vi "VisionX-1LOOP-Main.vi"(8 "ErrI":errorcluster) -> (0 "ErrO":errorcluster)   [LabVIEW 2020]
uses:
  <vilib>/vision/Measure.llb/Straight Edge Options.ctl
  <vilib>/vision/Measure.llb/Straight Edge Process.ctl
  <vilib>/vision/Image Controls.llb/IMAQ Image.ctl
  <vilib>/vision/Measure.llb/Edge Options.ctl
  <vilib>/vision/Measure.llb/Edge Polarity.ctl
  <vilib>/vision/NI_Vision_Development_Module.lvlib
panel:
  out "Pass?":bool
  out "Liquied Level":dbl format="%.2f"
  in  "Line Fit Options":T1={"Number of Lines"=1, "Type"=enum."Best Edge Rake", "Min. Score"=10.0, "Max. Score"=1000.0, "Orientation"=0.0, "Angle Range"=45.0, "Angle Tolerance"=1.0, "Step Size"=7, "Min. SNR (db)"=0.0, "Min. Points (%)"=25.0, "Hough Iterations"=5} {"Min. Points (%)" min=0.0 max=100.0; "Min. SNR (db)" min=0.0; "Max. Score" min=0.0 max=1024.0; "Min. Score" min=0.0 max=1024.0 step=1.0}
  out "Image":T3(plugin-control)
  in  "Next":bool
  in  "Exit":bool
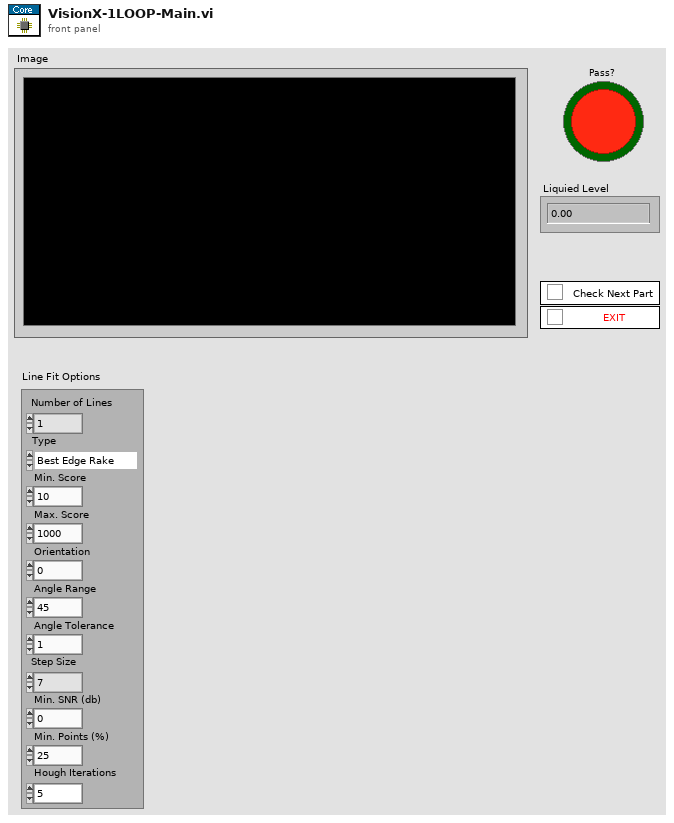
[diagram p1: front panel]
types:
  T1 = typedef "Straight Edge Options.ctl" = cluster{"Number of Lines":i32, "Type":T2, "Min. Score":dbl, "Max. Score":dbl, "Orientation":dbl, "Angle Range":dbl, "Angle Tolerance":dbl, "Step Size":u32, "Min. SNR (db)":dbl, "Min. Points (%)":dbl, "Hough Iterations":i32}
  T2 = typedef "Straight Edge Process.ctl" = enum32{"First Edge Rake", "Best Edge Rake", "Hough Edge Rake", "First Edge Projection", "Best Edge Projection"}
  T3 = typedef "IMAQ Image.ctl" = refnum<image>
  T4 = typedef "IMAQ Rectangle" = cluster{"Left":i32, "Top":i32, "Right":i32, "Bottom":i32, "Rotation":dbl}
  T5 = cluster{"Point1":cluster{"X":sgl, "Y":sgl}, "Point2":cluster{"X":sgl, "Y":sgl}}
  T6 = typedef "IMAQ Coordinate System" = cluster{"Reference System":cluster{"Origin":cluster{"X":sgl, "Y":sgl}, "Angle (deg)":sgl, "Axis Reference":u32}, "Measurement System":cluster{"Origin":cluster{"X":sgl, "Y":sgl}, "Angle (deg)":sgl, "Axis Reference":u32}}
  T7 = cluster{"Src":T3, "Dst":T3, "Parts":string[], "RefCoord":T6, "MsrCoord":T6, "MsrROI":T4, "RefLine":cluster{"Point1":cluster{"X":sgl, "Y":sgl}, "Point2":cluster{"X":sgl, "Y":sgl}}}
  T8 = typedef "Edge Options.ctl" = cluster{"Edge Polarity":T9, "Kernel Size":u32, "Width":u32, "Minimum Edge Strength":sgl, "Interpolation Type":enum32{"Zero Order", "Bilinear", "Quadratic", "Cubic", "Bilinear Fixed"}, "Data Processing Method":enum32{"Average", "Median"}}
  T9 = typedef "Edge Polarity.ctl" = u32
  T10 = cluster{"Direction":u16, "Primary Edge Options":T8, "Secondary Edge Options":T8, "Show Search Area":bool, "Show Search Lines":bool, "Show Edges Found":bool, "Show Result":bool, "Search Area Color":u32, "Search Lines Color":u32, "Edge Locations Color":u32, "Result Color":u32, "Overlay Group Name":string}
  T11 = typedef "ROI Descriptor" = cluster{"Global Rectangle":i32[], "Contours":cluster{"ID":enum32{"External", "Internal"}, "Type":u32, "Coordinates":i32[]}[]}
  T12 = cluster{"Search Direction":u32, "Edge Options":T8, "Show Search Area":bool, "Show Search Lines":bool, "Show Edges Found":bool, "Show Result":bool, "Search Area Color":u32, "Search Lines Color":u32, "Edge Locations Color":u32, "Result Color":u32, "Overlay Group Name":string}
  T13 = cluster{"Point1 (Pixels)":cluster{"X":sgl, "Y":sgl}, "Point2 (Pixels)":cluster{"X":sgl, "Y":sgl}, "Point1 (Real-World)":cluster{"X":sgl, "Y":sgl}, "Point2 (Real-World)":cluster{"X":sgl, "Y":sgl}, "Angle (Pixel)":dbl, "Angle (Real-World)":dbl, "Score":dbl, "Straightness":dbl, "Average SNR (db)":dbl, "Calibration Valid":bool}[]
  T14 = cluster{"Point1 (Pixels)":cluster{"X":sgl, "Y":sgl}, "Point2 (Pixels)":cluster{"X":sgl, "Y":sgl}, "Point1 (Real-World)":cluster{"X":sgl, "Y":sgl}, "Point2 (Real-World)":cluster{"X":sgl, "Y":sgl}, "Angle (Pixel)":dbl, "Angle (Real-World)":dbl, "Score":dbl, "Straightness":dbl, "Average SNR (db)":dbl, "Calibration Valid":bool}
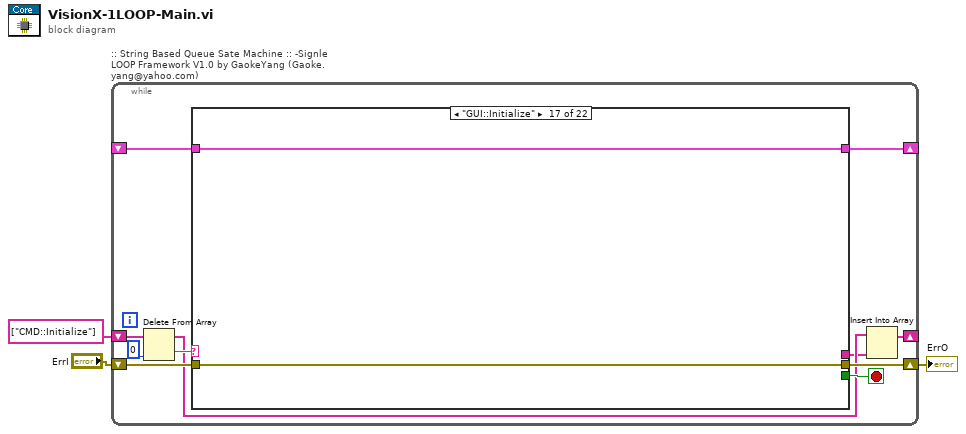
[diagram p0: block diagram]
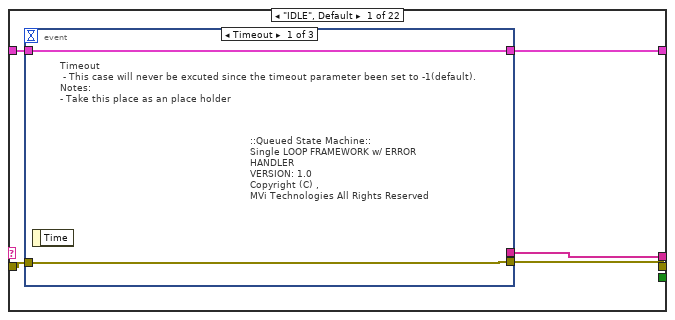
[diagram p2: hidden frame]
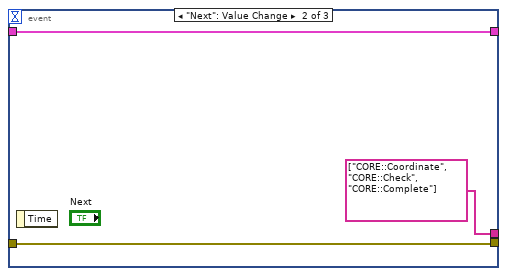
[diagram p3: hidden frame]
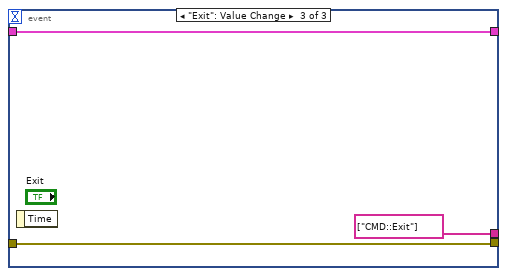
[diagram p4: hidden frame]
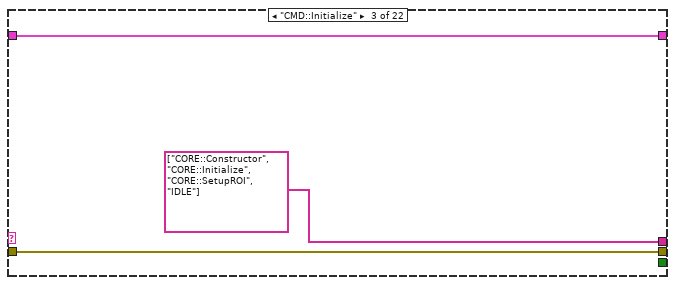
[diagram p6: hidden frame]
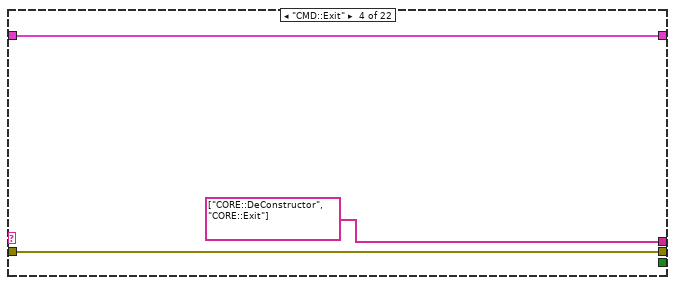
[diagram p7: hidden frame]
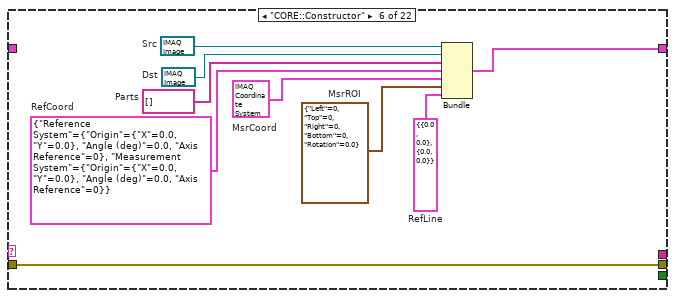
[diagram p9: hidden frame]
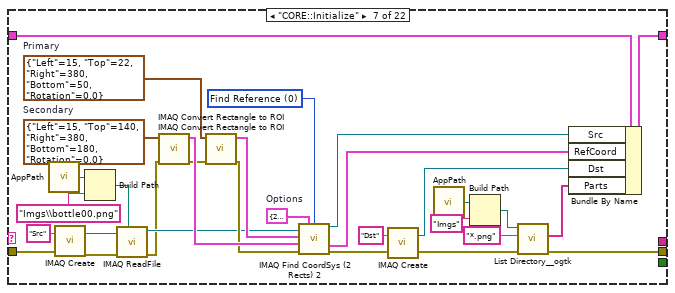
[diagram p10: hidden frame]
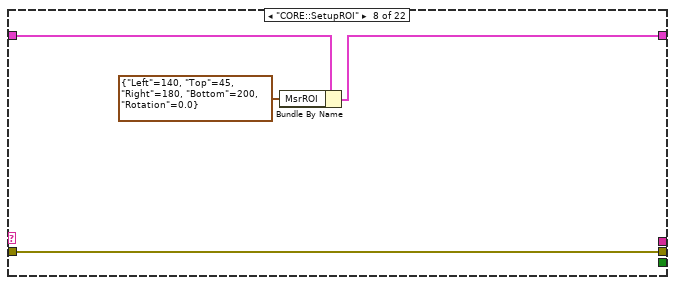
[diagram p11: hidden frame]
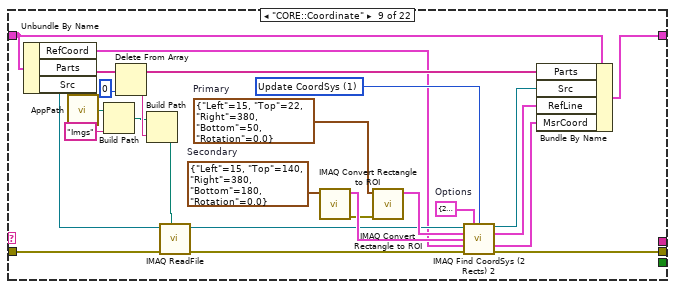
[diagram p12: hidden frame]
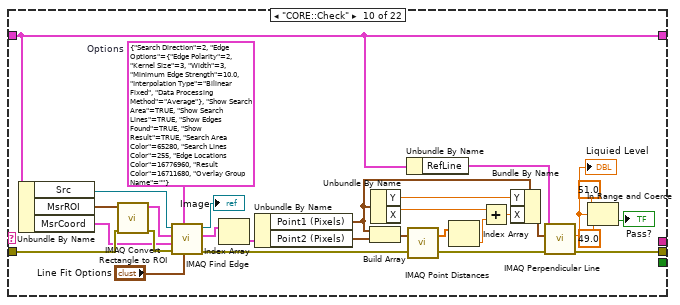
[diagram p13: hidden frame]
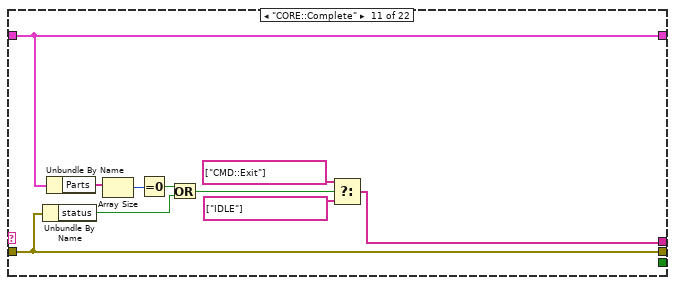
[diagram p14: hidden frame]
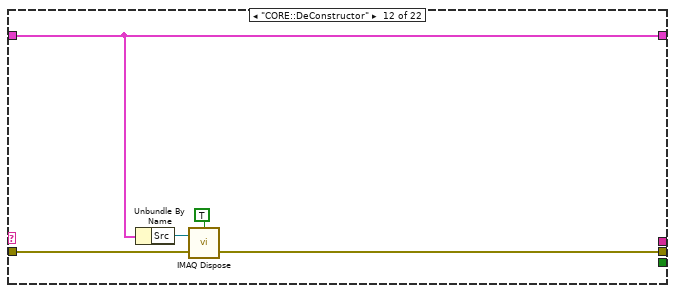
[diagram p15: hidden frame]
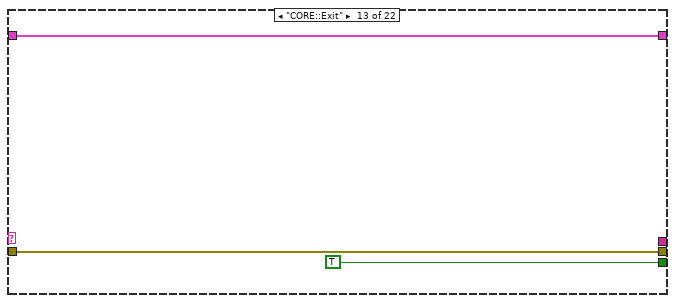
[diagram p16: hidden frame]
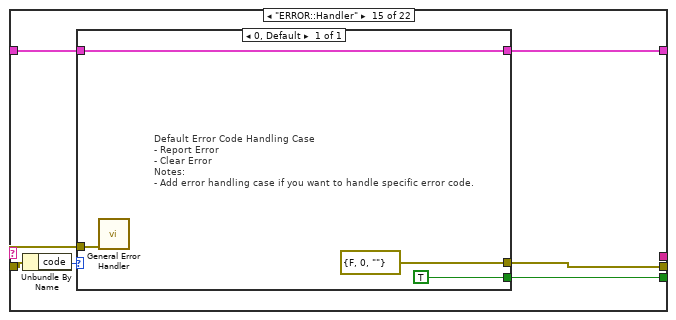
[diagram p18: hidden frame]
diagram:
  n1 = while ":: String Based Queue Sate Machine :: -Signle LOOP Framework V1.0 by GaokeYang (Gaoke.yang@yahoo.com)" {
    shift-right: [w11] -> w3
    shift-left: "ErrI" -> [w9]
    shift-right: [w13] -> _
    shift-left: _ -> [w12]
    shift-right: [w4] -> _
    shift-left: string[] ["CMD::Initialize"] -> [w10]
    stop <- w14 stop-if-true
    n2 = Delete From Array(array=w10, index=0) -> (deleted portion=w8:string, array with subset deleted=w6:string[])  [unwired: 1 in]
    n3 = case shown="\"GUI::Initialize\"" w8 {
      tunnel: [w18 w29 w31 w34 w37 w45 w70 w78 w89 w114 w142 w150 w152 w156 w159 w167 w169 w171 w174 w176 w178 w179] -> w11
      tunnel: [_ _ _ _ _ _ _ _ _ _ _ _ TRUE _ w158 _ _ _ _ _ _ _] -> w14
      tunnel: w9 -> [w19 w29 w31 w34 w37 w45 w72 w78 w104 w135 w142 w151 w152 w156 w157 w167 w169 w171 w174 w176 w178 w179]
      tunnel: [w16 w28 w32 w35 w36 w46 w75 w81 w101 w113 w143 w149 w153 w155 w160 w168 w170 w172 w173 w175 w177 w180] -> w13
      tunnel: w12 -> [w17 w28 w32 w35 w36 _ w76 w80 w102 w113 w143 w149 w153 w155 w161 w168 w170 w172 w173 w175 w177 w180]
      tunnel: [w15 _ string[] ["CORE::Constructor", "CORE::Initialize", "CORE::SetupROI", "IDLE"] string[] ["CORE::DeConstructor", "CORE::Exit"] _ _ _ _ _ _ w144 _ _ _ _ _ _ _ _ _ _ _] -> w5
      frame "IDLE", Default {
        n4 = event shown="[0] Timeout" {
          selector: _ -> [_ _ _]
          dyn-events: _ -> [_ _ _]
          timeout: _ -> [_ _ _]
          tunnel: [w21 w24 w27] -> w18
          tunnel: w19 -> [w21 w24 w27]
          tunnel: [w20 w23 w26] -> w16
          tunnel: w17 -> [w20 w23 w26]
          tunnel: [_ string[] ["CORE::Coordinate", "CORE::Check", "CORE::Complete"] string[] ["CMD::Exit"]] -> w15
          event Timeout {
            # "Timeout\n - This case will never be excuted since the timeout parameter been set to -1(default).\nNotes:\n- Take this place as an place holder"
            # "::Queued State Machine::\nSingle LOOP FRAMEWORK w/ ERROR HANDLER\nVERSION: 1.0\nCopyright (C) ,\nMVi Technologies All Rights Reserved"
            n5 = event-data() -> ()  [unwired: 1 in, 1 out]
          }
          event "Next": Value Change {
            n6 = event-data() -> ()  [unwired: 1 in, 1 out]
          }
          event "Exit": Value Change {
            n7 = event-data() -> ()  [unwired: 1 in, 1 out]
          }
        }
      }
      frame "-------- Commands ---------" {
      }
      frame "CMD::Initialize" {
      }
      frame "CMD::Exit" {
      }
      frame "------------ Core ------------" {
      }
      frame "CORE::Constructor" {
        w38 = T5 {"Point1"={"X"=0.0, "Y"=0.0}, "Point2"={"X"=0.0, "Y"=0.0}}  # RefLine
        w39 = T4 {"Left"=0, "Top"=0, "Right"=0, "Bottom"=0, "Rotation"=0.0}  # MsrROI
        w40 = T6 {"Reference System"={"Origin"={"X"=0.0, "Y"=0.0}, "Angle (deg)"=0.0, "Axis Reference"=0}, "Measurement System"={"Origin"={"X"=0.0, "Y"=0.0}, "Angle (deg)"=0.0, "Axis Reference"=0}}  # MsrCoord
        w41 = T6 {"Reference System"={"Origin"={"X"=0.0, "Y"=0.0}, "Angle (deg)"=0.0, "Axis Reference"=0}, "Measurement System"={"Origin"={"X"=0.0, "Y"=0.0}, "Angle (deg)"=0.0, "Axis Reference"=0}}  # RefCoord
        w44 = T3 refnum  # Dst
        w43 = string[] []  # Parts
        w42 = T3 refnum  # Src
        n8 = Bundle("Src"=w42, "Dst"=w44, "Parts"=w43, "RefCoord"=w41, "MsrCoord"=w40, "MsrROI"=w39, "RefLine"=w38) -> (w46:T7)  [unwired: 1 in]
      }
      frame "CORE::Initialize" {
        w62 = T4 {"Left"=15, "Top"=140, "Right"=380, "Bottom"=180, "Rotation"=0.0}  # Secondary
        w63 = T4 {"Left"=15, "Top"=22, "Right"=380, "Bottom"=50, "Rotation"=0.0}  # Primary
        w61 = T10 {"Direction"=2, "Primary Edge Options"={"Edge Polarity"=0, "Kernel Size"=3, "Width"=3, "Minimum Edge Strength"=10.0, "Interpolation Type"=enum."Bilinear Fixed", "Data Processing Method"=enum."Average"}, "Secondary Edge Options"={"Edge Polarity"=0, "Kernel Size"=3, "Width"=3, "Minimum Edge Strength"=10.0, "Interpolation Type"=enum."Bilinear Fixed", "Data Processing Method"=enum."Average"}, "Show Search Area"=TRUE, "Show Search Lines"=TRUE, "Show Edges Found"=TRUE, "Show Result"=TRUE, "Search Area Color"=65280, "Search Lines Color"=255, "Edge Locations Color"=14811391, "Result Color"=16711704, "Overlay Group Name"=""}  # Options
        w65 = u16 0 items=["Find Reference", "Update CoordSys"] ("Mode")
        n9 = call "AppPath.vi"() -> ("AppPath"=w52:path)
        n10 = call "IMAQ Create"("Image Name"="Src", "error in (no error)"=w72) -> ("New Image"=w74:T3, "error out"=w73:errorcluster)  [unwired: 3 in]
        n11 = Build Path(base path=w52, name or relative path="Imgs\\bottle00.png") -> (appended path=w50:path)
        n12 = call "IMAQ ReadFile"("File Path"=w50, "error in (no error)"=w73, "Image"=w74) -> ("error out"=w56:errorcluster, "Image Out"=w57:T3)  [unwired: 4 in, 3 out]
        n13 = call "IMAQ Convert Rectangle to ROI"("error in (no error)"=w56, "Rectangle"=w62) -> ("error out"=w60:errorcluster, "ROI Descriptor"=w64:T11)  [unwired: 7 in]
        n14 = call "IMAQ Convert Rectangle to ROI"("error in (no error)"=w60, "Rectangle"=w63) -> ("error out"=w59:errorcluster, "ROI Descriptor"=w58:T11)  [unwired: 7 in]
        n15 = call "IMAQ Find CoordSys (2 Rects) 2"("Image"=w57, "Options"=w61, "Mode"=w65, "Primary ROI Descriptor"=w58, "Secondary ROI Descriptor"=w64, "error in (no error)"=w59) -> ("Image Out"=w54:T3, "Coordinate System Out"=w53:T6, "error out"=w55:errorcluster)  [unwired: 5 in, 2 out]
        n16 = call "IMAQ Create"("Image Name"="Dst", "error in (no error)"=w55) -> ("New Image"=w67:T3, "error out"=w68:errorcluster)  [unwired: 3 in]
        n17 = call "AppPath.vi"() -> ("AppPath"=w48:path)
        n18 = Build Path(base path=w48, name or relative path="Imgs") -> (appended path=w47:path)
        n19 = call "List Directory__ogtk.vi"("error in (no error)"=w68, "pattern"="*.png", "directory path"=w47) -> ("error out"=w70:errorcluster, "file names"=w66:string[])  [unwired: 1 in, 2 out]
        n20 = Bundle By Name(cluster=w76, "Src"=w54, "RefCoord"=w53, "Dst"=w67, "Parts"=w66) -> (w75:T7)
      }
      frame "CORE::SetupROI" {
        n21 = Bundle By Name(cluster=w80, "MsrROI"=T4 {"Left"=140, "Top"=45, "Right"=180, "Bottom"=200, "Rotation"=0.0} ("Rectangle")) -> (w81:T7)
      }
      frame "CORE::Coordinate" {
        w95 = T4 {"Left"=15, "Top"=140, "Right"=380, "Bottom"=180, "Rotation"=0.0}  # Secondary
        w96 = T4 {"Left"=15, "Top"=22, "Right"=380, "Bottom"=50, "Rotation"=0.0}  # Primary
        w94 = T10 {"Direction"=2, "Primary Edge Options"={"Edge Polarity"=0, "Kernel Size"=3, "Width"=3, "Minimum Edge Strength"=10.0, "Interpolation Type"=enum."Bilinear Fixed", "Data Processing Method"=enum."Average"}, "Secondary Edge Options"={"Edge Polarity"=0, "Kernel Size"=3, "Width"=3, "Minimum Edge Strength"=10.0, "Interpolation Type"=enum."Bilinear Fixed", "Data Processing Method"=enum."Average"}, "Show Search Area"=TRUE, "Show Search Lines"=TRUE, "Show Edges Found"=TRUE, "Show Result"=TRUE, "Search Area Color"=65280, "Search Lines Color"=255, "Edge Locations Color"=14811391, "Result Color"=16711704, "Overlay Group Name"=""}  # Options
        w98 = u16 1 items=["Find Reference", "Update CoordSys"] ("Mode")
        n22 = Unbundle By Name(w102) -> ("RefCoord"=w87:T6, "Parts"=w100:string[], "Src"=w99:T3)
        n23 = call "AppPath.vi"() -> ("AppPath"=w84:path)
        n24 = Build Path(base path=w84, name or relative path="Imgs") -> (appended path=w83:path)
        n25 = Delete From Array(array=w100, index=0) -> (deleted portion=w106:string, array with subset deleted=w103:string[])  [unwired: 1 in]
        n26 = Build Path(base path=w83, name or relative path=w106) -> (appended path=w105:path)
        n27 = call "IMAQ ReadFile"("File Path"=w105, "error in (no error)"=w104, "Image"=w99) -> ("error out"=w91:errorcluster, "Image Out"=w90:T3)  [unwired: 4 in, 3 out]
        n28 = call "IMAQ Convert Rectangle to ROI"("Rectangle"=w95) -> ("error out"=w93:errorcluster, "ROI Descriptor"=w97:T11)  [unwired: 8 in]
        n29 = call "IMAQ Convert Rectangle to ROI"("error in (no error)"=w93, "Rectangle"=w96) -> ("ROI Descriptor"=w92:T11)  [unwired: 7 in, 1 out]
        n30 = call "IMAQ Find CoordSys (2 Rects) 2"("Image"=w90, "Options"=w94, "Mode"=w98, "Primary ROI Descriptor"=w92, "Secondary ROI Descriptor"=w97, "Coordinate System In"=w87, "error in (no error)"=w91) -> ("Image Out"=w88:T3, "Main Axis"=w86:T5, "Coordinate System Out"=w85:T6, "error out"=w89:errorcluster)  [unwired: 4 in, 1 out]
        n31 = Bundle By Name(cluster=w102, "Parts"=w103, "Src"=w88, "RefLine"=w86, "MsrCoord"=w85) -> (w101:T7)
      }
      frame "CORE::Check" {
        w129 = T12 {"Search Direction"=2, "Edge Options"={"Edge Polarity"=2, "Kernel Size"=3, "Width"=3, "Minimum Edge Strength"=10.0, "Interpolation Type"=enum."Bilinear Fixed", "Data Processing Method"=enum."Average"}, "Show Search Area"=TRUE, "Show Search Lines"=TRUE, "Show Edges Found"=TRUE, "Show Result"=TRUE, "Search Area Color"=65280, "Search Lines Color"=255, "Edge Locations Color"=16776960, "Result Color"=16711680, "Overlay Group Name"=""}  # Options
        n32 = Unbundle By Name(w113) -> ("Src"=w136:T3, "MsrROI"=w133:T4, "MsrCoord"=w131:T6)
        n33 = call "IMAQ Convert Rectangle to ROI"("error in (no error)"=w135, "Rectangle"=w133) -> ("error out"=w134:errorcluster, "ROI Descriptor"=w132:T11)  [unwired: 7 in]
        n34 = call "IMAQ Find Edge"("Line Fit Options"="Line Fit Options", "Options"=w129, "error in (no error)"=w134, "Coordinate System"=w131, "ROI Descriptor"=w132, "Image"=w136) -> ("error out"=w124:errorcluster, "Straight Edges"=w127:T13, "Image Out"=→"Image":T3)  [unwired: 2 in, 1 out]
        n35 = Index Array(array=w127) -> (element=w126:T14)  [unwired: 1 in]
        n36 = Unbundle By Name(w126) -> ("Point1 (Pixels)"=w117:cluster{"X":sgl, "Y":sgl}, "Point2 (Pixels)"=w116:cluster{"X":sgl, "Y":sgl})
        n37 = Build Array(w117, w116) -> (w125:cluster{"X":sgl, "Y":sgl}[])
        n38 = Unbundle By Name(w117) -> ("Y"=w120:sgl, "X"=w123:sgl)
        n39 = Unbundle By Name(w113) -> ("RefLine"=w112:T5)
        n40 = call "IMAQ Point Distances"("Points"=w125, "error in (no error)"=w124) -> ("Distances"=w122:sgl[], "error out"=w115:errorcluster)  [unwired: 3 in]
        n41 = Index Array(array=w122) -> (element=w121:sgl)  [unwired: 1 in]
        n42 = Add(x=w123, y=w121) -> (x+y=w119:sgl)
        n43 = Bundle By Name(cluster=w117, "Y"=w120, "X"=w119) -> (w118:cluster{"X":sgl, "Y":sgl})
        n44 = call "IMAQ Perpendicular Line"("error in (no error)"=w115, "Point"=w118, "Line"=w112) -> ("error out"=w114:errorcluster, "Distance"=w111:dbl)  [unwired: 6 in, 1 out]
        "Liquied Level" <- w111
        n45 = In Range and Coerce(upper limit=51.0, x=w111, lower limit=49.0) -> (In Range?=→"Pass?":bool)  [unwired: 1 out]
      }
      frame "CORE::Complete" {
        n46 = Unbundle By Name(w142) -> ("status"=w138:bool)
        n47 = Unbundle By Name(w143) -> ("Parts"=w141:string[])
        n48 = Array Size(array=w141) -> (size(s)=w140:i32)
        n49 = Equal To 0?(x=w140) -> (x = 0?=w139:bool)
        n50 = Or(x=w139, y=w138) -> (x .or. y?=w137:bool)
        n51 = Select(t=string[] ["CMD::Exit"], s=w137, f=string[] ["IDLE"]) -> (s? t:f=w144:string[])
      }
      frame "CORE::DeConstructor" {
        n52 = Unbundle By Name(w149) -> ("Src"=w148:T3)
        n53 = call "IMAQ Dispose"("All Images? (No)"=TRUE, "Image"=w148, "error in (no error)"=w151) -> ("error out"=w150:errorcluster)  [unwired: 3 in]
      }
      frame "CORE::Exit" {
      }
      frame "-------- Error Handle--------" {
      }
      frame "ERROR::Handler" {
        n54 = Unbundle By Name(w157) -> ("code"=w162:i32)
        n55 = case shown="0, Default" w162 {
          tunnel: [w166] -> w160
          tunnel: w161 -> [w166]
          tunnel: [errorcluster {"status"=FALSE, "code"=0, "source"=""} ("error out")] -> w159
          tunnel: [TRUE] -> w158
          tunnel: w157 -> [w164]
          frame 0, Default {
            # "Default Error Code Handling Case\n- Report Error\n- Clear Error \nNotes:\n- Add error handling case if you want to handle specific error code."
            n56 = call <vilib>:"General Error Handler.vi"("error in (no error)"=w164) -> ()  [unwired: 10 in, 5 out]
          }
        }
      }
      frame "------------  GUI  ------------" {
      }
      frame "GUI::Initialize" {
      }
      frame "GUI::SetCusor" {
      }
      frame "GUI::SetMenu" {
      }
      frame "------------ USER -----------" {
      }
      frame "USER::Case1" {
      }
      frame "USER::Case2" {
      }
    }
    n57 = Insert Into Array(array=w6, new element=w5) -> (w4:string[])  [unwired: 1 in]
  }
  "ErrO" <- w3
